vi "Simple Add.vi"() -> ()   [LabVIEW 2018]
panel:
  in  "y 2":dbl
  out "x+y":dbl
  in  "x":dbl
  in  "y":dbl
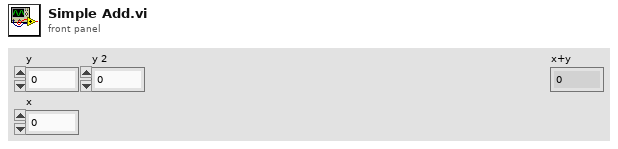
[diagram p1: front panel]
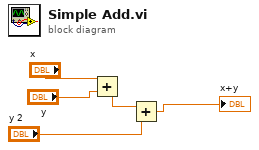
[diagram p0: block diagram]
diagram:
  n1 = Add(x="x", y="y") -> (x+y=w3:dbl)
  n2 = Add(x=w3, y="y 2") -> (x+y=→"x+y":dbl)
